vi "Custom User Scripting For New Override VI.vi"(8 "error in":errorcluster, 11 "VI Refnum in":refnum<vi>) -> (0 "error out":errorcluster)   [LabVIEW 2020]
doc: "When \"New >> VI For Override...\" is used to create a VI, this subVI will be invoked if the VI is created successfully after all other work to create the VI has been completed. Users may edit this subVI to add any instructions they wish for customizations of the newly generated VI."
uses:
  <vilib>/Utility/miscctls.llb/LVRectTypeDef.ctl
  <vilib>/regexp/Match Regular Expression.xnode
panel:
  out "error out 2":errorcluster
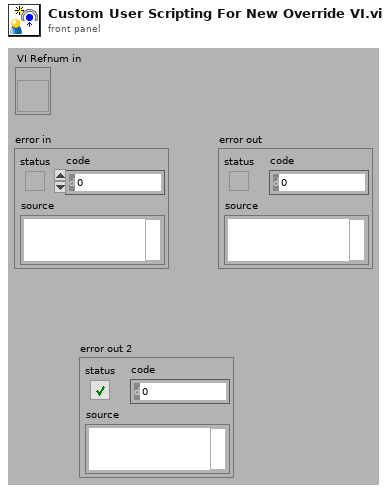
[diagram p1: front panel]
types:
  T1 = typedef "LVRectTypeDef.ctl" = cluster{"Left":i16, "Top":i16, "Right":i16, "Bottom":i16}
  T2 = cluster{"Class In":refnum<vi>, "Class Out":refnum<vi>, "Error In":refnum<vi>, "Error Out":refnum<vi>, "Other In":refnum<vi>[], "Other Out":refnum<vi>[]}
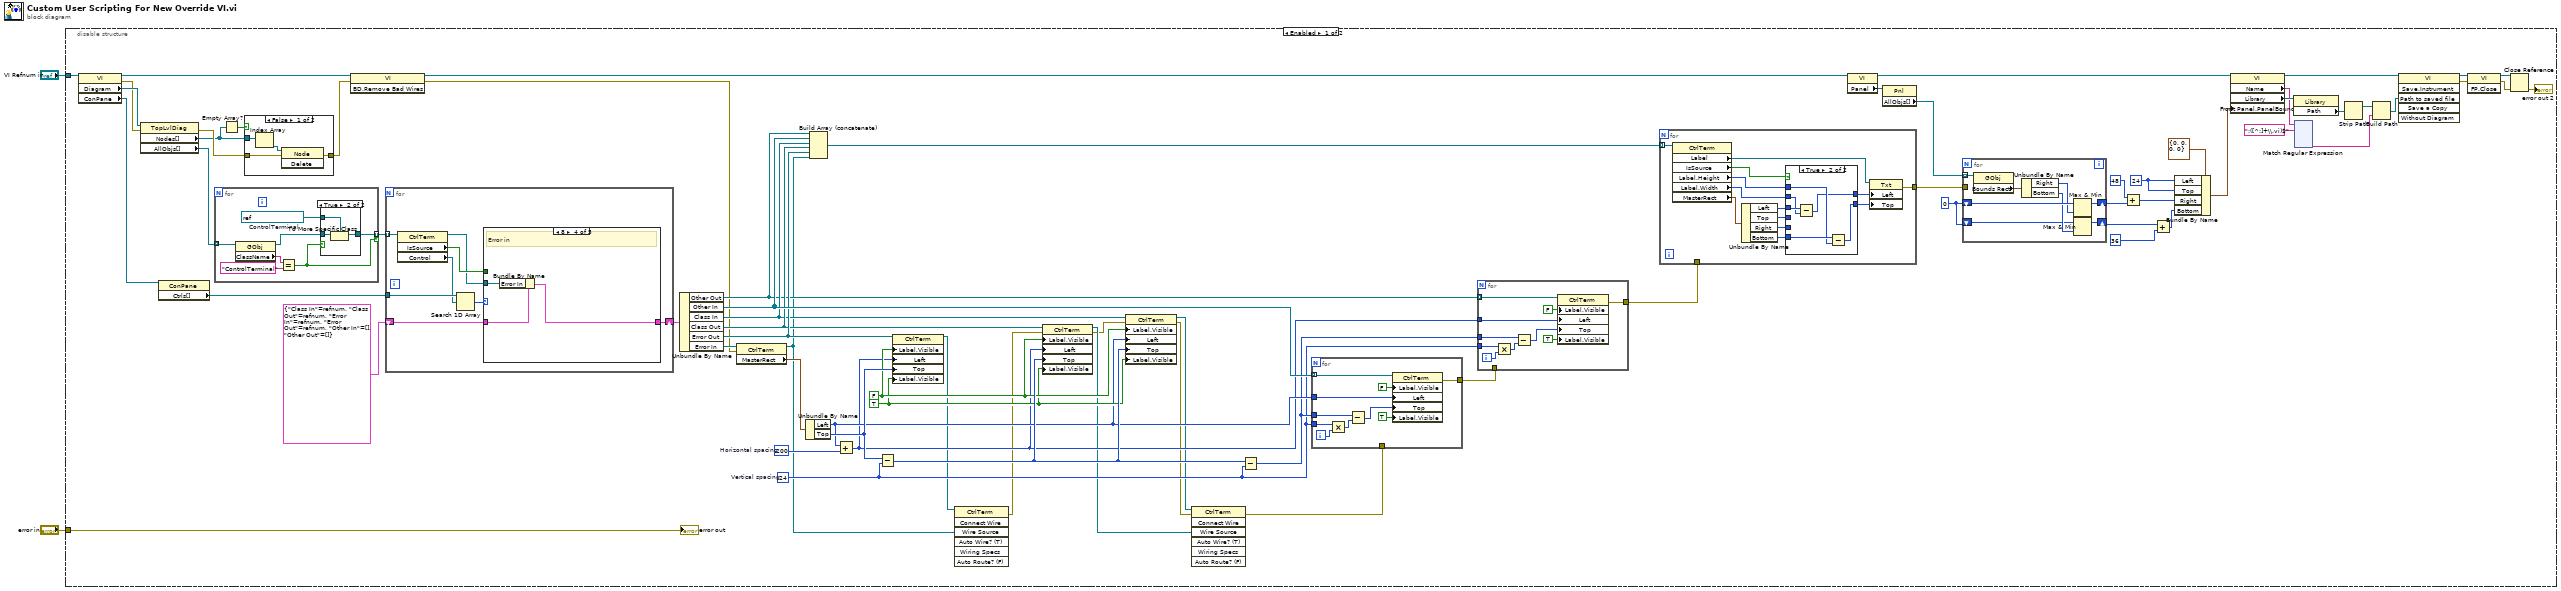
[diagram p0: block diagram]
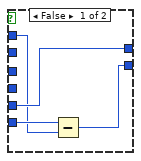
[diagram p3: hidden frame]
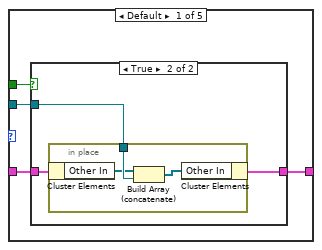
[diagram p4: hidden frame]
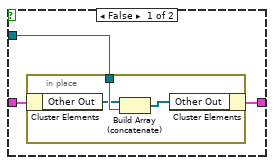
[diagram p5: hidden frame]
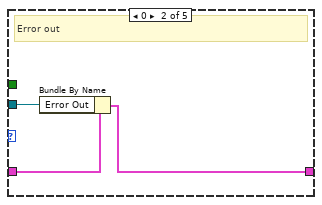
[diagram p6: hidden frame]
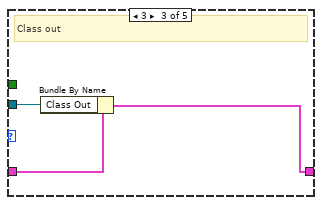
[diagram p7: hidden frame]
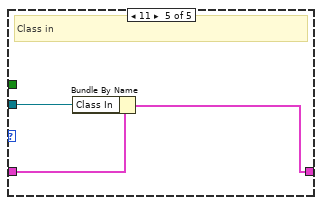
[diagram p8: hidden frame]
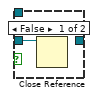
[diagram p9: hidden frame]
diagram:
  n1 = disable-structure shown="Enabled" {
    disable-tunnel: "error in" -> [w71 _]
    disable-tunnel: "VI Refnum in" -> [w70 _]
    frame Enabled {
      w15 = i16 24 ("x")
      w23 = i16 0 ("Right")
      w52 = TRUE ("Label.Visible")
      w53 = FALSE ("Label.Visible")
      w47 = 24  # Vertical spacing
      w63 = 200  # Horizontal spacing
      n2 = property class="VI"(reference=w70) -> (reference out=w26:refnum<vi>, error out=w68:errorcluster, "Diagram"=w69:refnum<vi>, "ConPane"=w41:refnum<vi>)  [unwired: 1 in]
      n3 = property class="TopLvlDiag"(reference=w69, error in=w68) -> (error out=w72:errorcluster, "Nodes[]"=w3:refnum<vi>[], "AllObjs[]"=w42:refnum<vi>[])  [unwired: 1 out]
      n4 = property class="ConPane"(reference=w41) -> ("Ctrls[]"=w66:refnum<vi>[])  [unwired: 1 in, 2 out]
      n5 = for {
        tunnel: w42 -> [w161] mode=indexing
        tunnel: [w156] -> w67 mode=indexing if=w155
        w157 = refnum<vi> refnum  # ControlTerminal
        n6 = property class="GObj"(reference=w161) -> (reference out=w158:refnum<vi>, "ClassName"=w160:string)  [unwired: 1 in, 1 out]
        n7 = Equal?(x=w160, y="ControlTerminal") -> (x = y?=w155:bool)
        n8 = case shown="True" w155 {
          tunnel: w158 -> [w162 w165]
          tunnel: w157 -> [_ w164]
          tunnel: [_ w163] -> w156
          frame False {
            n9 = Close Reference(reference=w162) -> ()  [unwired: 1 in, 1 out]
          }
          frame True {
            n10 = To More Specific Class(target class=w164, reference=w165) -> (specific class reference=w163:refnum<vi>)  [unwired: 1 in, 1 out]
          }
        }
      }
      n11 = Empty Array?(array=w3) -> (empty?=w4:bool)
      n12 = case shown="False" w4 {
        tunnel: w72 -> [w76 w77]
        tunnel: w3 -> [w75 _]
        tunnel: [w73 w77] -> w10
        frame False {
          n13 = Index Array(array=w75) -> (element=w74:refnum<vi>)  [unwired: 1 in]
          n14 = invoke class="Node" method="Delete"(reference=w74, error in=w76) -> (error out=w73:errorcluster)  [unwired: 1 in, 2 out]
        }
        frame True {
        }
      }
      n15 = invoke class="VI" method="BD.Remove Bad Wires"(reference=w26, error in=w10) -> (reference out=w11:refnum<vi>, error out=w9:errorcluster)  [unwired: 1 in, 1 out]
      n16 = for {
        tunnel: w67 -> [w126] mode=indexing
        tunnel: w66 -> [w125]
        shift-right: [w120] -> w64
        shift-left: T2 {"Class In"=refnum, "Class Out"=refnum, "Error In"=refnum, "Error Out"=refnum, "Other In"=[], "Other Out"=[]} -> [w123]
        n17 = property class="CtrlTerm"(reference=w126) -> (reference out=w119:refnum<vi>, "IsSource"=w121:bool, "Control"=w122:refnum<vi>)  [unwired: 1 in, 1 out]
        n18 = Search 1D Array(1D array=w125, element=w122) -> (index of element=w124:i32)  [unwired: 1 in]
        n19 = case shown="8" w124 {
          tunnel: w123 -> [w129 w145 w148 w151 w154]
          tunnel: w119 -> [w128 w144 w147 w150 w153]
          tunnel: w121 -> [w130 _ _ _ _]
          tunnel: [w127 w143 w146 w149 w152] -> w120
          frame Default {
            n20 = case shown="True" w130 {
              tunnel: w129 -> [w133 w138]
              tunnel: w128 -> [w132 w139]
              tunnel: [w131 w137] -> w127
              frame False {
                n21 = in-place {
                  in-place-border: w132 -> [w136]
                  n22 = in-place-cluster #1(w133) -> ("Other Out"=w135:refnum<vi>[])
                  n23 = Build Array (concatenate)(w135, w136) -> (w134:refnum<vi>[])
                  n24 = in-place-cluster #1("Other Out"=w134) -> (w131:T2)
                }
              }
              frame True {
                n25 = in-place {
                  in-place-border: w139 -> [w142]
                  n26 = in-place-cluster #2(w138) -> ("Other In"=w141:refnum<vi>[])
                  n27 = Build Array (concatenate)(w141, w142) -> (w140:refnum<vi>[])
                  n28 = in-place-cluster #2("Other In"=w140) -> (w137:T2)
                }
              }
            }
          }
          frame 0 {
            # "Error out"
            n29 = Bundle By Name(cluster=w145, "Error Out"=w144) -> (w143:T2)
          }
          frame 3 {
            # "Class out"
            n30 = Bundle By Name(cluster=w148, "Class Out"=w147) -> (w146:T2)
          }
          frame 8 {
            # "Error in"
            n31 = Bundle By Name(cluster=w151, "Error In"=w150) -> (w149:T2)
          }
          frame 11 {
            # "Class in"
            n32 = Bundle By Name(cluster=w154, "Class In"=w153) -> (w152:T2)
          }
        }
      }
      n33 = Unbundle By Name(w64) -> ("Other Out"=w50:refnum<vi>[], "Other In"=w62:refnum<vi>[], "Class In"=w55:refnum<vi>, "Class Out"=w56:refnum<vi>, "Error Out"=w58:refnum<vi>, "Error In"=w60:refnum<vi>)
      n34 = property class="CtrlTerm"(reference=w60, error in=w9) -> (reference out=w46:refnum<vi>, "MasterRect"=w59:T1)  [unwired: 1 out]
      n35 = Unbundle By Name(w59) -> ("Left"=w51:i16, "Top"=w57:i16)
      n36 = Build Array (concatenate)(w50, w62, w55, w56, w58, w46) -> (w61:refnum<vi>[])
      n37 = Add(x=w51, y=w63) -> (x+y=w49:i32)
      n38 = Subtract(x=w57, y=w47) -> (x-y=w54:i32)
      n39 = property class="CtrlTerm"(reference=w58, "Label.Visible"=w53, "Left"=w49, "Top"=w57, "Label.Visible"=w52) -> (reference out=w45:refnum<vi>)  [unwired: 1 in, 1 out]
      n40 = invoke class="CtrlTerm" method="Connect Wire"(reference=w45, "Wire Source"=w46) -> (error out=w40:errorcluster)  [unwired: 5 in, 6 out]
      n41 = property class="CtrlTerm"(reference=w56, error in=w40, "Label.Visible"=w53, "Left"=w49, "Top"=w54, "Label.Visible"=w52) -> (reference out=w43:refnum<vi>, error out=w39:errorcluster)
      n42 = property class="CtrlTerm"(reference=w55, error in=w39, "Label.Visible"=w53, "Left"=w51, "Top"=w54, "Label.Visible"=w52) -> (reference out=w44:refnum<vi>, error out=w38:errorcluster)
      n43 = invoke class="CtrlTerm" method="Connect Wire"(reference=w44, error in=w38, "Wire Source"=w43) -> (error out=w37:errorcluster)  [unwired: 4 in, 6 out]
      n44 = Subtract(x=w54, y=w47) -> (x-y=w48:i32)
      n45 = for {
        tunnel: w47 -> [w175]
        tunnel: w48 -> [w173]
        tunnel: w62 -> [w171] mode=indexing
        tunnel: w51 -> [w168]
        tunnel: w37 -> [_]
        tunnel: [w166] -> w36
        i -> [w174]
        n46 = Multiply(x=w175, y=w174) -> (x*y=w172:i32)
        n47 = Subtract(x=w173, y=w172) -> (x-y=w170:i32)
        n48 = property class="CtrlTerm"(reference=w171, "Label.Visible"=FALSE, "Left"=w168, "Top"=w170, "Label.Visible"=TRUE) -> (error out=w166:errorcluster)  [unwired: 1 in, 1 out]
      }
      n49 = for {
        tunnel: w47 -> [w95]
        tunnel: w48 -> [w93]
        tunnel: w50 -> [w91] mode=indexing
        tunnel: w49 -> [w88]
        tunnel: w36 -> [_]
        tunnel: [w86] -> w35
        i -> [w94]
        n50 = Multiply(x=w95, y=w94) -> (x*y=w92:i32)
        n51 = Subtract(x=w93, y=w92) -> (x-y=w90:i32)
        n52 = property class="CtrlTerm"(reference=w91, "Label.Visible"=FALSE, "Left"=w88, "Top"=w90, "Label.Visible"=TRUE) -> (error out=w86:errorcluster)  [unwired: 1 in, 1 out]
      }
      n53 = for {
        tunnel: w61 -> [w108] mode=indexing
        tunnel: w35 -> [_]
        tunnel: [w96] -> w25
        n54 = property class="CtrlTerm"(reference=w108) -> ("Label"=w107:refnum<vi>, "IsSource"=w105:bool, "Label.Height"=w104:u32, "Label.Width"=w103:u32, "MasterRect"=w106:T1)  [unwired: 1 in, 2 out]
        n55 = Unbundle By Name(w106) -> ("Left"=w102:i16, "Top"=w101:i16, "Right"=w100:i16, "Bottom"=w99:i16)
        n56 = case shown="True" w105 {
          tunnel: w104 -> [w110 w117]
          tunnel: w103 -> [_ w115]
          tunnel: w102 -> [_ w116]
          tunnel: w101 -> [_ _]
          tunnel: w100 -> [w112 _]
          tunnel: w99 -> [w111 w118]
          tunnel: [w112 w113] -> w98
          tunnel: [w109 w114] -> w97
          frame False {
            n57 = Subtract(x=w111, y=w110) -> (x-y=w109:u32)
          }
          frame True {
            n58 = Subtract(x=w116, y=w115) -> (x-y=w113:u32)
            n59 = Subtract(x=w118, y=w117) -> (x-y=w114:u32)
          }
        }
        n60 = property class="Txt"(reference=w107, "Left"=w98, "Top"=w97) -> (error out=w96:errorcluster)  [unwired: 1 in, 1 out]
      }
      n61 = property class="VI"(reference=w11) -> (reference out=w16:refnum<vi>, "Panel"=w27:refnum<vi>)  [unwired: 1 in, 1 out]
      n62 = property class="Pnl"(reference=w27) -> ("AllObjs[]"=w24:refnum<vi>[])  [unwired: 1 in, 2 out]
      n63 = for {
        tunnel: w25 -> [_]
        tunnel: w24 -> [w85] mode=indexing
        shift-right: [w82] -> w19
        shift-left: w23 -> [w83]
        shift-right: [w81] -> w20
        shift-left: w23 -> [w78]
        n64 = property class="GObj"(reference=w85) -> ("Bounds Rect"=w84:T1)  [unwired: 1 in, 2 out]
        n65 = Unbundle By Name(w84) -> ("Right"=w80:i16, "Bottom"=w79:i16)
        n66 = Max & Min(x=w83, y=w80) -> (max(x,y)=w82:i16)  [unwired: 1 out]
        n67 = Max & Min(x=w78, y=w79) -> (max(x,y)=w81:i16)  [unwired: 1 out]
      }
      n68 = Add(x=i16 48, y=w19) -> (x+y=w18:i16)
      n69 = Add(x=w20, y=i16 36 ("x")) -> (x+y=w17:i16)
      n70 = Bundle By Name(cluster=T1 {"Left"=0, "Top"=0, "Right"=0, "Bottom"=0} ("Front Panel Window:Panel Bounds"), "Left"=w15, "Top"=w15, "Right"=w18, "Bottom"=w17) -> (w21:T1)
      n71 = property class="VI"(reference=w16, "Front Panel.PanelBounds"=w21) -> ("Name"=w30:string, "Library"=w34:refnum<vi>)  [unwired: 1 in, 2 out]
      n72 = property class="Library"(reference=w34) -> ("Path"=w33:path)  [unwired: 1 in, 2 out]
      n73 = xnode "Match Regular Expression"("input string"=w30, "regular expression"=":([^:]+\\.vi)$") -> ("submatch 1"=w28:string)  [unwired: 4 in, 5 out]
      n74 = Strip Path(path=w33) -> (stripped path=w32:path)  [unwired: 1 out]
      n75 = Build Path(base path=w32, name or relative path=w28) -> (appended path=w31:path)
      n76 = invoke class="VI" method="Save.Instrument"(reference=w16, "Path to saved file"=w31) -> (reference out=w12:refnum<vi>, error out=w6:errorcluster)  [unwired: 4 in, 4 out]
      n77 = invoke class="VI" method="FP.Close"(reference=w12, error in=w6) -> (reference out=w8:refnum<vi>, error out=w7:errorcluster)  [unwired: 1 in, 1 out]
      n78 = Close Reference(reference=w8, error in (no error)=w7) -> (error out=→"error out 2":errorcluster)
      "error out" <- w71
    }
    frame Disabled {
    }
  }
